vi "Read Anything.vi"(0 "refnum":T1, 5 "user parameter references in":refnum<vi>[](array[refnum]), 11 "error in":errorcluster, 12 "additional information":string) -> (4 "refnum out":T1, 15 "error out":errorcluster)   [LabVIEW 2023, in "TLB` InstStu GPlugin Template.lvlib" / "{TMPL} TLB`.lvclass"]
uses:
  {TMPL} TLB`.lvclass
  {TMPL} TLB`.lvclass/{TMPL} TLB`.ctl
  <vilib>/Utility/config.llb/NI_LVConfig.lvlib
  <vilib>/Utility/config.llb/Read Key (String).vi
  <vilib>/Utility/config.llb/Config Data RefNum.ctl
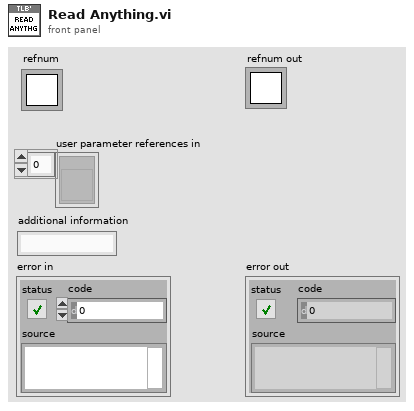
[diagram p1: front panel]
types:
  T1 = typedef "NI_LVConfig.lvlib/Config Data RefNum.ctl" = refnum<k1>
  T2 = typedef "LVNumericRepresentation.ctl" = enum32{"Extended Precision", "Double Precision", "Single Precision", "Long", "Word", "Byte", "Unsigned Long", "Unsigned Word", "Unsigned Byte", "Complex Extended", "Complex Double", "Complex Single", "Quad", "Unsigned Quad", "Fixed-Point"}
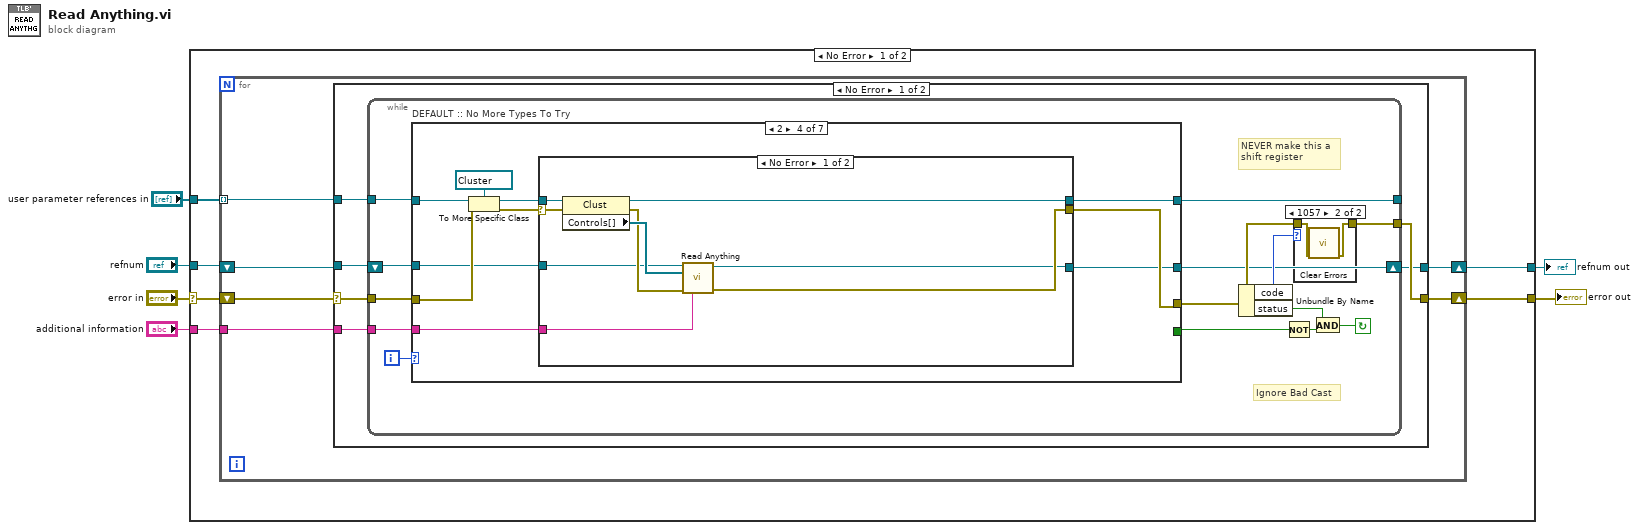
[diagram p0: block diagram]
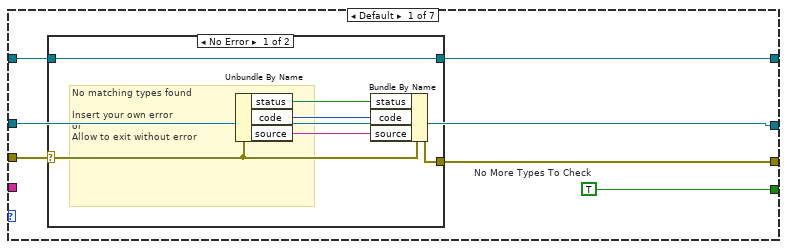
[diagram p2: hidden frame]
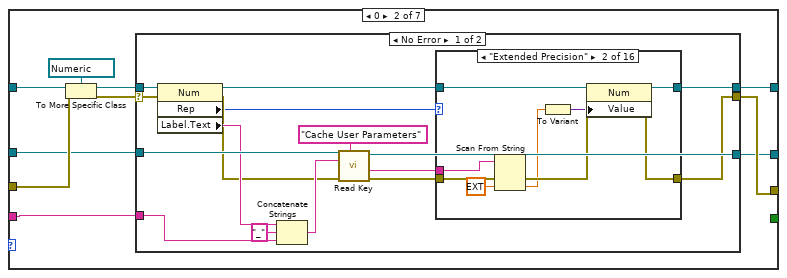
[diagram p4: hidden frame]
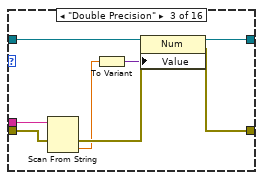
[diagram p6: hidden frame]
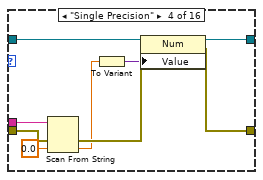
[diagram p7: hidden frame]
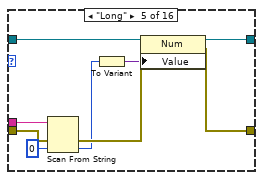
[diagram p8: hidden frame]
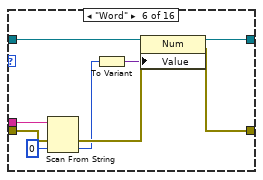
[diagram p9: hidden frame]
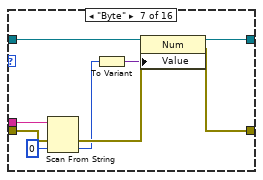
[diagram p10: hidden frame]
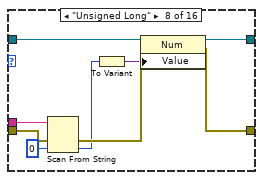
[diagram p11: hidden frame]
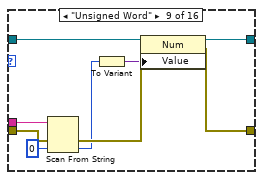
[diagram p12: hidden frame]
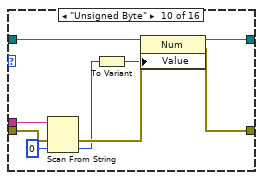
[diagram p13: hidden frame]
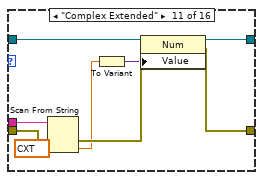
[diagram p14: hidden frame]
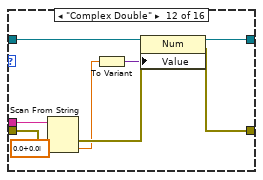
[diagram p15: hidden frame]
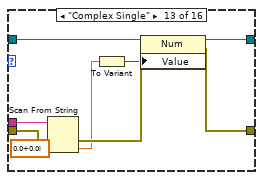
[diagram p16: hidden frame]
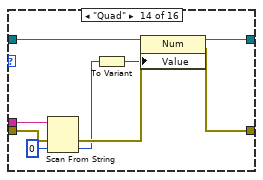
[diagram p17: hidden frame]
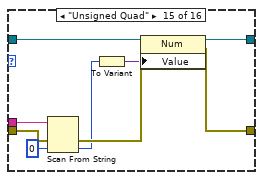
[diagram p18: hidden frame]
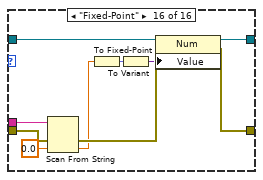
[diagram p19: hidden frame]
diagram:
  n1 = case shown="No Error" "error in" {
    selector: "error in" -> [w10 w378]
    tunnel: "user parameter references in" -> [w12 _]
    tunnel: [w11 w378] -> w4
    tunnel: "refnum" -> [w9 w377]
    tunnel: [w8 w377] -> w2
    tunnel: "additional information" -> [w7 _]
    frame No Error {
      n2 = for {
        tunnel: w12 -> [w16] mode=indexing
        shift-right: [w18] -> w11
        shift-left: w10 -> [w17]
        shift-right: [w15] -> w8
        shift-left: w9 -> [w14]
        tunnel: w7 -> [w13]
        n3 = case shown="No Error" w17 {
          selector: w17 -> [w23 w376]
          tunnel: w16 -> [w24 _]
          tunnel: [w22 w376] -> w18
          tunnel: w14 -> [w21 w375]
          tunnel: [w20 w375] -> w15
          tunnel: w13 -> [w19 _]
          frame No Error {
            n4 = while {
              tunnel: w24 -> [w34]
              tunnel: w23 -> [w32]
              tunnel: [w29] -> _
              tunnel: [w28] -> w22
              shift-right: [w26] -> w20
              shift-left: w21 -> [w27]
              tunnel: w19 -> [w25]
              i -> [w33]
              stop <- w35 continue-if-true
              # "NEVER make this a\nshift register"
              # "Ignore Bad Cast"
              n5 = case "DEFAULT :: No More Types To Try" shown="2" w33 {
                tunnel: w32 -> [w41 w62 w228 w257 w278 w319 w347]
                tunnel: w34 -> [w42 w60 w226 w255 w276 w317 w345]
                tunnel: [w43 w56 w222 w251 w272 w313 w341] -> w29
                tunnel: [w40 w57 w223 w252 w273 w314 w342] -> w31
                tunnel: [w44 _ _ _ _ _ _] -> w30
                tunnel: w27 -> [w39 w55 w221 w250 w271 w312 w340]
                tunnel: [w39 w54 w220 w249 w270 w311 w339] -> w26
                tunnel: w25 -> [_ w53 w219 w248 _ w310 w338]
                frame Default {
                  w44 = TRUE  # No More Types To Check
                  n6 = case shown="No Error" w41 {
                    selector: w41 -> [w48 w51]
                    tunnel: [w50 w52] -> w43
                    tunnel: w42 -> [w50 w52]
                    tunnel: [w49 w51] -> w40
                    frame No Error {
                      # "No matching types found\n\nInsert your own error \nor\nAllow to exit without error"
                      n7 = Unbundle By Name(w48) -> ("status"=w47:bool, "code"=w46:i32, "source"=w45:string)
                      n8 = Bundle By Name(cluster=w48, "status"=w47, "code"=w46, "source"=w45) -> (w49:errorcluster)
                    }
                    frame Error {
                      # "No matching types found\n\nAllow this non-typecast error to propogate through without modification"
                    }
                  }
                }
                frame 0 {
                  n9 = To More Specific Class(target class=refnum<vi> refnum ("Waveform Chart"), reference=w60, error in=w62) -> (specific class reference=w59:refnum<vi>, error out=w58:errorcluster)
                  n10 = case shown="No Error" w58 {
                    selector: w58 -> [w77 w218]
                    tunnel: w59 -> [w78 w217]
                    tunnel: [w63 w218] -> w57
                    tunnel: [w65 w217] -> w56
                    tunnel: w55 -> [w75 w216]
                    tunnel: [w74 w216] -> w54
                    tunnel: w53 -> [w71 _]
                    frame No Error {
                      n11 = property class="Num"(reference=w78, error in=w77) -> (reference out=w66:refnum<vi>, error out=w69:errorcluster, "Rep"=w67:T2, "Label.Text"=w73:string)
                      n12 = Concatenate Strings(w73, "_" ("string"), w71) -> (w72:string)
                      n13 = call-poly <vilib>:"Read Key.vi"("section"="Cache User Parameters", "error in (no error)"=w69, "key"=w72, "refnum"=w75) -> ("error out"=w64:errorcluster, "value"=w68:string, "refnum out"=w74:T1)  [unwired: 4 in, 1 out]
                      n14 = case shown="\"Extended Precision\"" w67 {
                        tunnel: w68 -> [_ w81 w95 w104 w113 w122 w131 w140 w149 w158 w167 w176 w185 w194 w203 w213]
                        tunnel: w66 -> [w80 w86 w97 w106 w115 w124 w133 w142 w151 w160 w169 w178 w187 w196 w205 w215]
                        tunnel: [w80 w85 w96 w105 w114 w123 w132 w141 w150 w159 w168 w177 w186 w195 w204 w214] -> w65
                        tunnel: w64 -> [w79 w83 w94 w103 w112 w121 w130 w139 w148 w157 w166 w175 w184 w193 w202 w212]
                        tunnel: [w79 w84 w92 w101 w110 w119 w128 w137 w146 w155 w164 w173 w182 w191 w200 w210] -> w63
                        frame Default {
                        }
                        frame "Extended Precision" {
                          n15 = Scan From String(input string=w81, error in=w83, default 1=ext 0.0 ("default value 1")) -> (error out=w89:errorcluster, output 1=w88:ext)  [unwired: 2 in, 2 out]
                          n16 = To Variant(anything=w88) -> (Variant=w87:variant)
                          n17 = property class="Num"(reference=w86, error in=w89, "Value"=w87) -> (reference out=w85:refnum<vi>, error out=w84:errorcluster)
                        }
                        frame "Double Precision" {
                          n18 = Scan From String(input string=w95, error in=w94) -> (error out=w93:errorcluster, output 1=w91:dbl)  [unwired: 3 in, 2 out]
                          n19 = To Variant(anything=w91) -> (Variant=w90:variant)
                          n20 = property class="Num"(reference=w97, error in=w93, "Value"=w90) -> (reference out=w96:refnum<vi>, error out=w92:errorcluster)
                        }
                        frame "Single Precision" {
                          n21 = Scan From String(input string=w104, error in=w103, default 1=sgl 0.0 ("default value 1")) -> (error out=w102:errorcluster, output 1=w100:sgl)  [unwired: 2 in, 2 out]
                          n22 = To Variant(anything=w100) -> (Variant=w99:variant)
                          n23 = property class="Num"(reference=w106, error in=w102, "Value"=w99) -> (reference out=w105:refnum<vi>, error out=w101:errorcluster)
                        }
                        frame "Long" {
                          n24 = Scan From String(input string=w113, error in=w112, default 1=0 ("default value 1")) -> (error out=w111:errorcluster, output 1=w109:i32)  [unwired: 2 in, 2 out]
                          n25 = To Variant(anything=w109) -> (Variant=w108:variant)
                          n26 = property class="Num"(reference=w115, error in=w111, "Value"=w108) -> (reference out=w114:refnum<vi>, error out=w110:errorcluster)
                        }
                        frame "Word" {
                          n27 = Scan From String(input string=w122, error in=w121, default 1=i16 0 ("default value 1")) -> (error out=w120:errorcluster, output 1=w118:i16)  [unwired: 2 in, 2 out]
                          n28 = To Variant(anything=w118) -> (Variant=w117:variant)
                          n29 = property class="Num"(reference=w124, error in=w120, "Value"=w117) -> (reference out=w123:refnum<vi>, error out=w119:errorcluster)
                        }
                        frame "Byte" {
                          n30 = Scan From String(input string=w131, error in=w130, default 1=i8 0 ("default value 1")) -> (error out=w129:errorcluster, output 1=w127:i8)  [unwired: 2 in, 2 out]
                          n31 = To Variant(anything=w127) -> (Variant=w126:variant)
                          n32 = property class="Num"(reference=w133, error in=w129, "Value"=w126) -> (reference out=w132:refnum<vi>, error out=w128:errorcluster)
                        }
                        frame "Unsigned Long" {
                          n33 = Scan From String(input string=w140, error in=w139, default 1=u32 0 ("default value 1")) -> (error out=w138:errorcluster, output 1=w136:u32)  [unwired: 2 in, 2 out]
                          n34 = To Variant(anything=w136) -> (Variant=w135:variant)
                          n35 = property class="Num"(reference=w142, error in=w138, "Value"=w135) -> (reference out=w141:refnum<vi>, error out=w137:errorcluster)
                        }
                        frame "Unsigned Word" {
                          n36 = Scan From String(input string=w149, error in=w148, default 1=u16 0 ("default value 1")) -> (error out=w147:errorcluster, output 1=w145:u16)  [unwired: 2 in, 2 out]
                          n37 = To Variant(anything=w145) -> (Variant=w144:variant)
                          n38 = property class="Num"(reference=w151, error in=w147, "Value"=w144) -> (reference out=w150:refnum<vi>, error out=w146:errorcluster)
                        }
                        frame "Unsigned Byte" {
                          n39 = Scan From String(input string=w158, error in=w157, default 1=u8 0 ("default value 1")) -> (error out=w156:errorcluster, output 1=w154:u8)  [unwired: 2 in, 2 out]
                          n40 = To Variant(anything=w154) -> (Variant=w153:variant)
                          n41 = property class="Num"(reference=w160, error in=w156, "Value"=w153) -> (reference out=w159:refnum<vi>, error out=w155:errorcluster)
                        }
                        frame "Complex Extended" {
                          n42 = Scan From String(input string=w167, error in=w166, default 1=cxt 0.0+0.0i ("default value 1")) -> (error out=w165:errorcluster, output 1=w163:cxt)  [unwired: 2 in, 2 out]
                          n43 = To Variant(anything=w163) -> (Variant=w162:variant)
                          n44 = property class="Num"(reference=w169, error in=w165, "Value"=w162) -> (reference out=w168:refnum<vi>, error out=w164:errorcluster)
                        }
                        frame "Complex Double" {
                          n45 = Scan From String(input string=w176, error in=w175, default 1=cdb 0.0+0.0i ("default value 1")) -> (error out=w174:errorcluster, output 1=w172:cdb)  [unwired: 2 in, 2 out]
                          n46 = To Variant(anything=w172) -> (Variant=w171:variant)
                          n47 = property class="Num"(reference=w178, error in=w174, "Value"=w171) -> (reference out=w177:refnum<vi>, error out=w173:errorcluster)
                        }
                        frame "Complex Single" {
                          n48 = Scan From String(input string=w185, error in=w184, default 1=csg 0.0+0.0i ("default value 1")) -> (error out=w183:errorcluster, output 1=w181:csg)  [unwired: 2 in, 2 out]
                          n49 = To Variant(anything=w181) -> (Variant=w180:variant)
                          n50 = property class="Num"(reference=w187, error in=w183, "Value"=w180) -> (reference out=w186:refnum<vi>, error out=w182:errorcluster)
                        }
                        frame "Quad" {
                          n51 = Scan From String(input string=w194, error in=w193, default 1=i64 0 ("default value 1")) -> (error out=w192:errorcluster, output 1=w190:i64)  [unwired: 2 in, 2 out]
                          n52 = To Variant(anything=w190) -> (Variant=w189:variant)
                          n53 = property class="Num"(reference=w196, error in=w192, "Value"=w189) -> (reference out=w195:refnum<vi>, error out=w191:errorcluster)
                        }
                        frame "Unsigned Quad" {
                          n54 = Scan From String(input string=w203, error in=w202, default 1=u64 0 ("default value 1")) -> (error out=w201:errorcluster, output 1=w199:u64)  [unwired: 2 in, 2 out]
                          n55 = To Variant(anything=w199) -> (Variant=w198:variant)
                          n56 = property class="Num"(reference=w205, error in=w201, "Value"=w198) -> (reference out=w204:refnum<vi>, error out=w200:errorcluster)
                        }
                        frame "Fixed-Point" {
                          n57 = Scan From String(input string=w213, error in=w212, default 1=0.0 ("default value 1")) -> (error out=w211:errorcluster, output 1=w206:dbl)  [unwired: 2 in, 2 out]
                          n58 = To Fixed-Point(number=w206) -> (fixed-point=w207:fxp<+/-,32,16>)  [unwired: 1 in]
                          n59 = To Variant(anything=w207) -> (Variant=w209:variant)
                          n60 = property class="Num"(reference=w215, error in=w211, "Value"=w209) -> (reference out=w214:refnum<vi>, error out=w210:errorcluster)
                        }
                      }
                    }
                    frame Error {
                    }
                  }
                }
                frame 1 {
                  n61 = To More Specific Class(target class=refnum<vi> refnum ("Waveform Chart"), reference=w226, error in=w228) -> (specific class reference=w225:refnum<vi>, error out=w224:errorcluster)
                  n62 = case shown="No Error" w224 {
                    selector: w224 -> [w243 w247]
                    tunnel: w225 -> [w244 w246]
                    tunnel: [w229 w247] -> w223
                    tunnel: [w233 w246] -> w222
                    tunnel: w221 -> [w241 w245]
                    tunnel: [w240 w245] -> w220
                    tunnel: w219 -> [w236 _]
                    frame No Error {
                      n63 = property class="Path"(reference=w244, error in=w243) -> (reference out=w234:refnum<vi>, error out=w238:errorcluster, "Label.Text"=w239:string)
                      n64 = Concatenate Strings(w239, "_" ("string"), w236) -> (w237:string)
                      n65 = call-poly <vilib>:"Read Key.vi"("section"="Cache User Parameters", "error in (no error)"=w238, "key"=w237, "refnum"=w241) -> ("error out"=w230:errorcluster, "value"=w232:string, "refnum out"=w240:T1)  [unwired: 4 in, 1 out]
                      n66 = String To Path(string=w232) -> (path=w231:path)
                      n67 = property class="Path"(reference=w234, error in=w230, "Value"=w231) -> (reference out=w233:refnum<vi>, error out=w229:errorcluster)
                    }
                    frame Error {
                    }
                  }
                }
                frame 2 {
                  n68 = To More Specific Class(target class=refnum<vi> refnum ("Waveform Chart"), reference=w255, error in=w257) -> (specific class reference=w254:refnum<vi>, error out=w253:errorcluster)
                  n69 = case shown="No Error" w253 {
                    selector: w253 -> [w265 w269]
                    tunnel: w254 -> [w266 w268]
                    tunnel: [w261 w269] -> w252
                    tunnel: [w264 w268] -> w251
                    tunnel: w250 -> [w260 w267]
                    tunnel: [w259 w267] -> w249
                    tunnel: w248 -> [w258 _]
                    frame No Error {
                      n70 = property class="Clust"(reference=w266, error in=w265) -> (reference out=w264:refnum<vi>, error out=w262:errorcluster, "Controls[]"=w263:refnum<vi>[])
                      n71 = call "Read Anything.vi"("refnum"=w260, "user parameter references in"=w263, "error in"=w262, "additional information"=w258) -> ("refnum out"=w259:T1, "error out"=w261:errorcluster)  [unwired: 10 in]
                    }
                    frame Error {
                    }
                  }
                }
                frame 3 {
                  n72 = To More Specific Class(target class=refnum<vi> refnum ("Waveform Chart"), reference=w276, error in=w278) -> (specific class reference=w275:refnum<vi>, error out=w274:errorcluster)
                  n73 = case shown="No Error" w274 {
                    selector: w274 -> [w292 w309]
                    tunnel: w275 -> [w293 w308]
                    tunnel: [w291 w309] -> w273
                    tunnel: [w286 w308] -> w272
                    tunnel: w271 -> [w290 w307]
                    tunnel: [w289 w307] -> w270
                    frame No Error {
                      n74 = property class="Arr"(reference=w293, error in=w292) -> (reference out=w287:refnum<vi>, error out=w280:errorcluster, "Value"=w285:variant)
                      n75 = Build Array(variant ("type")) -> (w283:variant[])
                      n76 = Variant To Data(error in=w280, type=w283, Variant=w285) -> (data=w282:variant[], error out=w279:errorcluster)
                      n77 = Array Size(array=w282) -> (size(s)=w281:i32)
                      n78 = To Long Integer(number=w281) -> (32bit integer=w288:i32)
                      n79 = for {
                        N: w288 -> [_]
                        shift-right: [w306] -> w291
                        shift-left: w279 -> [w302]
                        shift-right: [w304] -> w289
                        shift-left: w290 -> [w305]
                        tunnel: w287 -> [w303]
                        tunnel: [w303] -> w286
                        i -> [w295]
                        n80 = Build Array(w295) -> (w301:i32[])
                        n81 = To Unsigned Long Integer(number=w301) -> (unsigned 32bit integer=w297:u32[])
                        n82 = property class="Arr"(reference=w303, error in=w302, "Index Values"=w297) -> (error out=w300:errorcluster, "Array Element"=w299:refnum<vi>)  [unwired: 1 out]
                        n83 = Format Into String(format string="(%d)", w295) -> (resulting string=w296:string)  [unwired: 2 in, 1 out]
                        n84 = Build Array(w299) -> (w298:refnum<vi>[])
                        n85 = call "Read Anything.vi"("refnum"=w305, "user parameter references in"=w298, "error in"=w300, "additional information"=w296) -> ("refnum out"=w304:T1, "error out"=w306:errorcluster)  [unwired: 10 in]
                      }
                    }
                    frame Error {
                    }
                  }
                }
                frame 4 {
                  n86 = To More Specific Class(target class=refnum<vi> refnum ("Waveform Chart"), reference=w317, error in=w319) -> (specific class reference=w316:refnum<vi>, error out=w315:errorcluster)
                  n87 = case shown="No Error" w315 {
                    selector: w315 -> [w333 w337]
                    tunnel: w316 -> [w334 w336]
                    tunnel: [w320 w337] -> w314
                    tunnel: [w323 w336] -> w313
                    tunnel: w312 -> [w331 w335]
                    tunnel: [w330 w335] -> w311
                    tunnel: w310 -> [w326 _]
                    frame No Error {
                      n88 = property class="Str"(reference=w334, error in=w333) -> (reference out=w324:refnum<vi>, error out=w328:errorcluster, "Label.Text"=w329:string)
                      n89 = Concatenate Strings(w329, "_" ("string"), w326) -> (w327:string)
                      n90 = call-poly <vilib>:"Read Key.vi"("section"="Cache User Parameters", "error in (no error)"=w328, "key"=w327, "refnum"=w331) -> ("error out"=w321:errorcluster, "value"=w322:string, "refnum out"=w330:T1)  [unwired: 4 in, 1 out]
                      n91 = property class="Str"(reference=w324, error in=w321, "Value"=w322) -> (reference out=w323:refnum<vi>, error out=w320:errorcluster)
                    }
                    frame Error {
                    }
                  }
                }
                frame 5 {
                  n92 = To More Specific Class(target class=refnum<vi> refnum ("Waveform Chart"), reference=w345, error in=w347) -> (specific class reference=w344:refnum<vi>, error out=w343:errorcluster)
                  n93 = case shown="No Error" w343 {
                    selector: w343 -> [w363 w371]
                    tunnel: w344 -> [w364 w370]
                    tunnel: [w349 w371] -> w342
                    tunnel: [w352 w370] -> w341
                    tunnel: w340 -> [w355 w369]
                    tunnel: [w361 w369] -> w339
                    tunnel: w338 -> [w358 _]
                    frame No Error {
                      n94 = property class="Bool"(reference=w364, error in=w363) -> (reference out=w353:refnum<vi>, error out=w356:errorcluster, "Label.Text"=w360:string)
                      n95 = Concatenate Strings(w360, "_" ("string"), w358) -> (w359:string)
                      n96 = call-poly <vilib>:"Read Key.vi"("section"="Cache User Parameters", "error in (no error)"=w356, "key"=w359, "refnum"=w355) -> ("error out"=w350:errorcluster, "value"=w354:string, "refnum out"=w361:T1)  [unwired: 4 in, 1 out]
                      n97 = To Lower Case(string=w354) -> (all lower case string=w351:string)
                      n98 = case shown="\"true\"" w351 {
                        tunnel: [w365 w367] -> w348
                        frame "false", Default {
                          n99 = To Variant(anything=FALSE) -> (Variant=w365:variant)
                        }
                        frame "true" {
                          n100 = To Variant(anything=TRUE) -> (Variant=w367:variant)
                        }
                      }
                      n101 = property class="Bool"(reference=w353, error in=w350, "Value"=w348) -> (reference out=w352:refnum<vi>, error out=w349:errorcluster)
                    }
                    frame Error {
                    }
                  }
                }
              }
              n102 = Unbundle By Name(w31) -> ("code"=w36:i32, "status"=w37:bool)
              n103 = Not(x=w30) -> (.not. x?=w38:bool)
              n104 = case shown="1057" w36 {
                tunnel: [w372 w374] -> w28
                tunnel: w31 -> [w372 w373]
                frame Default {
                }
                frame 1057 {
                  n105 = call <vilib>:"Clear Errors.vi"("error in (no error)"=w373) -> ("error out"=w374:errorcluster)  [unwired: 5 in, 1 out]
                }
              }
              n106 = And(x=w37, y=w38) -> (x .and. y?=w35:bool)
            }
          }
          frame Error {
          }
        }
      }
    }
    frame Error {
    }
  }
  "error out" <- w4
  "refnum out" <- w2
